vi "FlatToRichpumploop_GetValveResult.vi"(5 "OutputClusterType":T1, 11 "InputCluster":T3) -> (3 "OutputCluster":T1)   [LabVIEW 2024, in "pumploop_client.lvlib"]
uses:
  pumploop_client.lvlib
  pumploop_GetValveResult_Flat.ctl
  pumploop_Valves_Flat.ctl
  pumploop_GetValveResult.ctl
  pumploop_Valves.ctl
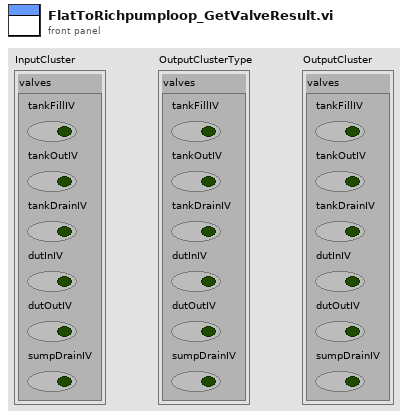
[diagram p1: front panel]
types:
  T1 = typedef "pumploop_client.lvlib/pumploop_GetValveResult.ctl" = cluster{"valves":T2}
  T2 = typedef "pumploop_client.lvlib/pumploop_Valves.ctl" = cluster{"tankFillIV":bool, "tankOutIV":bool, "tankDrainIV":bool, "dutInIV":bool, "dutOutIV":bool, "sumpDrainIV":bool}
  T3 = typedef "pumploop_client.lvlib/pumploop_GetValveResult_Flat.ctl" = cluster{"valves":T4}
  T4 = typedef "pumploop_client.lvlib/pumploop_Valves_Flat.ctl" = cluster{"tankFillIV":bool, "tankOutIV":bool, "tankDrainIV":bool, "dutInIV":bool, "dutOutIV":bool, "sumpDrainIV":bool}
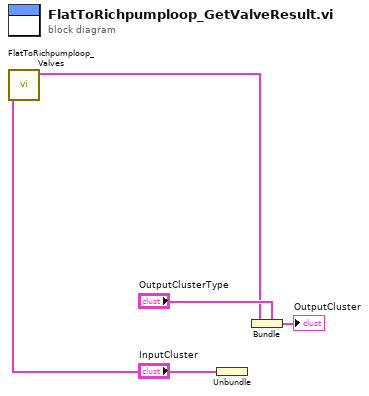
[diagram p0: block diagram]
diagram:
  n1 = Unbundle "Unbundle"("InputCluster") -> ("valves"=w2:T4)
  n2 = call "FlatToRichpumploop_Valves.vi"("InputCluster"=w2) -> ("OutputCluster"=w1:T2)  [unwired: 10 in]
  n3 = Bundle "Bundle"(cluster="OutputClusterType", "valves"=w1) -> (→"OutputCluster":T1)
